vi "Untitled 2.vi"   [LabVIEW 2011]
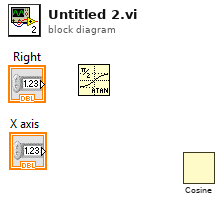
[diagram p0: block diagram]
diagram:
  n1 = Cosine() -> ()  [unwired: 1 in, 1 out]
